vi "Realback2.vi"() -> ()   [LabVIEW 2013]
uses:
  <vilib>/Utility/file.llb/Write To Spreadsheet File (DBL).vi
  <vilib>/Utility/file.llb/Read From Spreadsheet File (DBL).vi
panel:
  out "Output array":dbl[][](array[numeric])=[[211.6, 0.38780028612303014], [211.60999999999999, 0.3845669527896967], [211.62, 0.3657997138769633], [211.63, 0.3474805436337587], [211.64, 0.32995436337624834], [211.65, 0.3122437768240314], [211.66, 0.2951436337625158], [211.67, 0.2787942775393399], [211.68, 0.2629261802575091], [211.69, 0.24712174535049974], [211.7, 0.23246380543633732], [211.71, 0.21756866952789733], [211.72, 0.2032354792560812], [211.73, 0.18945178826895767], [211.74, 0.17619527896995957], [211.75, 0.16343619456366493], [211.76, 0.1512828326180282], [211.77, 0.13936108726752736], [211.78, 0.12796037195994514], [211.79, 0.11670128755365022], [211.8, 0.10619170243204774], [211.81, 0.09626437768240538], [211.82, 0.08718154506437926], [211.82999999999998, 0.07816609442060239], [211.84, 0.06949399141631024], [211.85, 0.06115035765379196], [211.85999999999999, 0.05409570815450693], [211.87, 0.04653447782546495], [211.88, 0.040030901287553614], [211.89, 0.034256080114449174], [211.9, 0.028719027181688065], [211.91, 0.023262804005722462], [211.92, 0.019033476394849768], [211.93, 0.015508154506437763], [211.94, 0.011468955650929882], [211.95, 0.008281545064377656], [211.96, 0.005692417739628017], [211.97, 0.0037329041487839517], [211.98, 0.0022765379113018377], [211.99, 0.0005326180257510675], [212.0, 0.0005386266094420548], [212.01, 0.001001144492131604], [212.02, 0.0015979971387696558], [212.03, 0.0031499284692417515], [212.04, 0.004863090128755342], [212.05, 0.006630185979971357], [212.06, 0.009368669527896977], [212.07, 0.012598998569384807], [212.08, 0.016054649499284653], [212.09, 0.020632474964234614], [212.1, 0.0254995708154506], [212.11, 0.030854792560801106], [212.12, 0.037168669527896915], [212.13, 0.043395278969957006], [212.14000000000001, 0.050058226037196306], [212.15, 0.05790472103004361], [212.16, 0.06554334763948602], [212.17000000000002, 0.07354535050071673], [212.18, 0.08245851216023044], [212.19, 0.09229155937053117], [212.2, 0.10267010014306345], [212.21, 0.11381888412017369], [212.22, 0.12524005722460899], [212.23, 0.13723304721030297], [212.24, 0.14960200286123287], [212.25, 0.1625593705293301], [212.26, 0.17595951359084663], [212.27, 0.19006294706724108], [212.28, 0.2049556509299012], [212.29, 0.22014062947067292], [212.3, 0.23593648068669504], [212.31, 0.25293133047210187], [212.32, 0.27017496423461923], [212.33, 0.28806266094420385], [212.34, 0.30654978540772254], [212.35, 0.3253447782546466], [212.36, 0.34475236051501806], [212.37, 0.36438998569384445], [212.38, 0.3852260371959913], [212.39000000000001, 0.4064221745350483], [212.4, 0.42819256080114376]]
  in  "# of data rows":i32=91
  out "Voffset":dbl=6.2433 format="%_5g"
  out "Vtune":dbl=0.935 format="%_5g"
  out "Volts":dbl=3.245 format="%_4g"
  out "Temp C":dbl=24.12 format="%_4g"
  in  "# skip":i32
  in  "# of sweeps":i32=700
  out "Spectrum #":i32=699
  out "Chars":i32=494328
  out "Fcen":dbl=212.0 format="%#_13g"
  out "# Data points":i32=81
  in  "Offset V":dbl=0.032 format="%#_3g"
  out "NMR Graph + Fit":cluster{dbl, dbl}[](graph)=[{211.6, 0.38780028612303014}, {211.60999999999999, 0.3845669527896967}, {211.62, 0.3657997138769633}, {211.63, 0.3474805436337587}, {211.64, 0.32995436337624834}, {211.65, 0.3122437768240314}, {211.66, 0.2951436337625158}, {211.67, 0.2787942775393399}, {211.68, 0.2629261802575091}, {211.69, 0.24712174535049974}, {211.7, 0.23246380543633732}, {211.71, 0.21756866952789733}, {211.72, 0.2032354792560812}, {211.73, 0.18945178826895767}, {211.74, 0.17619527896995957}, {211.75, 0.16343619456366493}, {211.76, 0.1512828326180282}, {211.77, 0.13936108726752736}, {211.78, 0.12796037195994514}, {211.79, 0.11670128755365022}, {211.8, 0.10619170243204774}, {211.81, 0.09626437768240538}, {211.82, 0.08718154506437926}, {211.82999999999998, 0.07816609442060239}, {211.84, 0.06949399141631024}, {211.85, 0.06115035765379196}, {211.85999999999999, 0.05409570815450693}, {211.87, 0.04653447782546495}, {211.88, 0.040030901287553614}, {211.89, 0.034256080114449174}, {211.9, 0.028719027181688065}, {211.91, 0.023262804005722462}, {211.92, 0.019033476394849768}, {211.93, 0.015508154506437763}, {211.94, 0.011468955650929882}, {211.95, 0.008281545064377656}, {211.96, 0.005692417739628017}, {211.97, 0.0037329041487839517}, {211.98, 0.0022765379113018377}, {211.99, 0.0005326180257510675}, {212.0, 0.0005386266094420548}, {212.01, 0.001001144492131604}, {212.02, 0.0015979971387696558}, {212.03, 0.0031499284692417515}, {212.04, 0.004863090128755342}, {212.05, 0.006630185979971357}, {212.06, 0.009368669527896977}, {212.07, 0.012598998569384807}, {212.08, 0.016054649499284653}, {212.09, 0.020632474964234614}, {212.1, 0.0254995708154506}, {212.11, 0.030854792560801106}, {212.12, 0.037168669527896915}, {212.13, 0.043395278969957006}, {212.14000000000001, 0.050058226037196306}, {212.15, 0.05790472103004361}, {212.16, 0.06554334763948602}, {212.17000000000002, 0.07354535050071673}, {212.18, 0.08245851216023044}, {212.19, 0.09229155937053117}, {212.2, 0.10267010014306345}, {212.21, 0.11381888412017369}, {212.22, 0.12524005722460899}, {212.23, 0.13723304721030297}, {212.24, 0.14960200286123287}, {212.25, 0.1625593705293301}, {212.26, 0.17595951359084663}, {212.27, 0.19006294706724108}, {212.28, 0.2049556509299012}, {212.29, 0.22014062947067292}, {212.3, 0.23593648068669504}, {212.31, 0.25293133047210187}, {212.32, 0.27017496423461923}, {212.33, 0.28806266094420385}, {212.34, 0.30654978540772254}, {212.35, 0.3253447782546466}, {212.36, 0.34475236051501806}, {212.37, 0.36438998569384445}, {212.38, 0.3852260371959913}, {212.39000000000001, 0.4064221745350483}, {212.4, 0.42819256080114376}]
  out "File size (bytes)":i32=509277
  out "File name":string="C:\\Users\\plm\\Desktop\\rssmt\\NMR3521123599.xls"
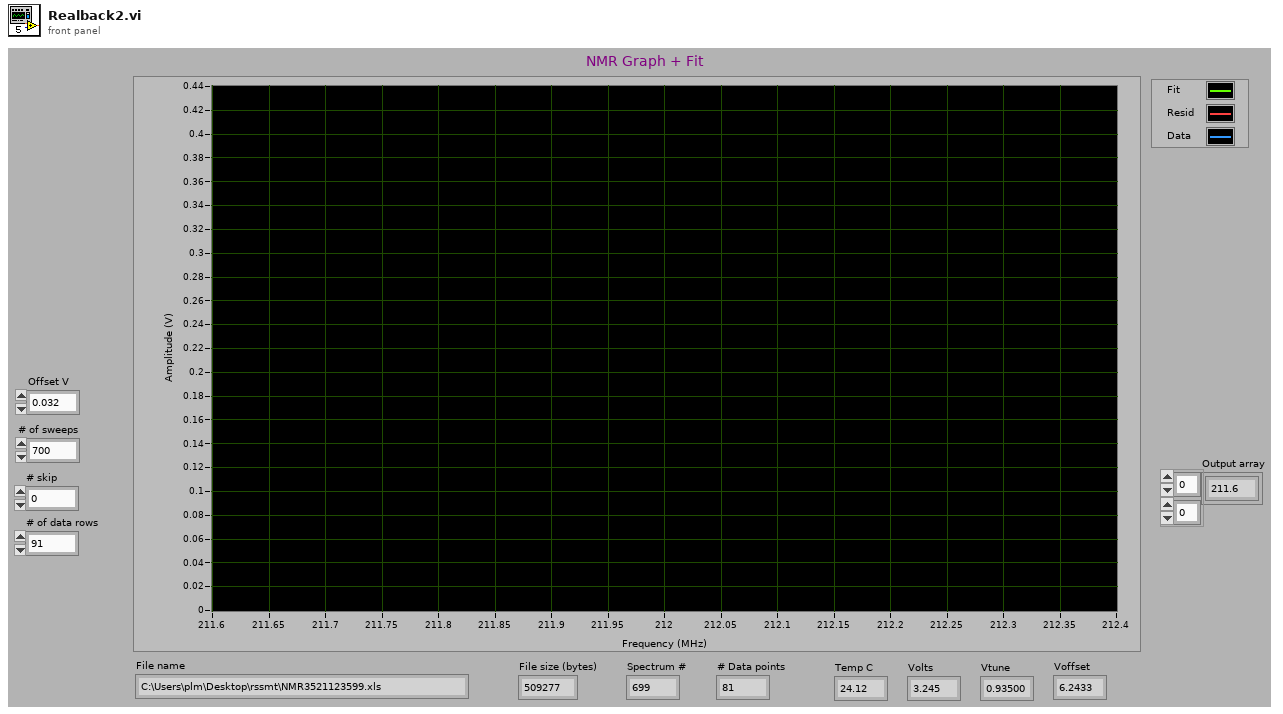
[diagram p1: front panel]
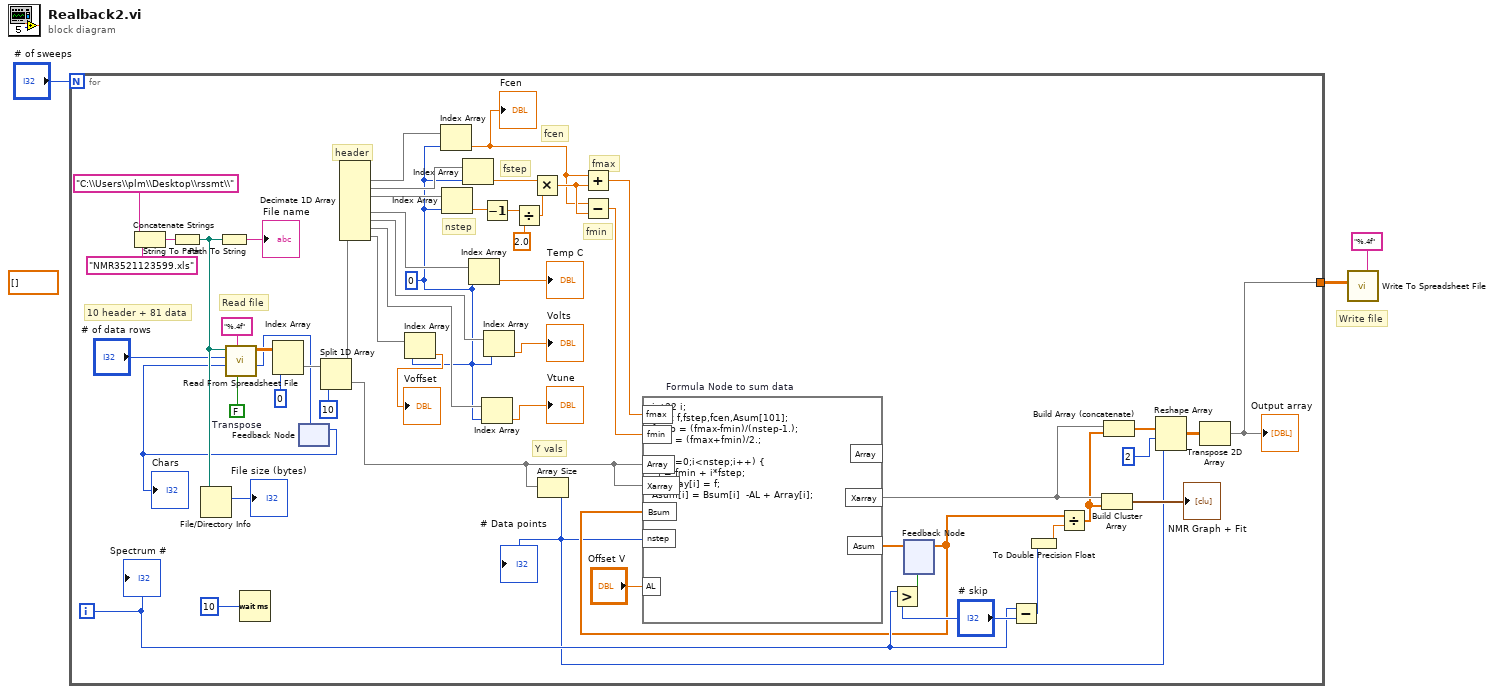
[diagram p0: block diagram]
diagram:
  (unwired) dbl[] []
  # "Write file"
  n1 = for {
    N: "# of sweeps" -> [_]
    tunnel: [w5] -> w1
    i -> [w26]
    w12 = 0
    w54 = FALSE  # Transpose
    # "10 header + 81 data"
    # "Read file"
    # "header"
    # "nstep"
    # "fstep"
    # "fcen"
    # "fmin"
    # "fmax"
    # "Y vals"
    n2 = Concatenate Strings "Concatenate Strings"("C:\\Users\\plm\\Desktop\\rssmt\\", "NMR3521123599.xls") -> (w57:string)
    n3 = String To Path(string=w57) -> (path=w53:path)
    n4 = File/Directory Info(path=w53) -> (size=→"File size (bytes)":i64)  [unwired: 1 in, 6 out]
    n5 = Path To String(path=w53) -> (string=→"File name":string)
    n6 = Wait (ms)(milliseconds to wait=10) -> ()  [unwired: 1 out]
    n7 = feedback #1() -> (w32:i32)  [unwired: 1 in]
    "Chars" <- w32
    n8 = call-poly <vilib>:"Read From Spreadsheet File.vi"("transpose (no:F)"=w54, "format (%.3f)"="%.4f", "start of read offset (chars.:0)"=w32, "number of rows (all:-1)"="# of data rows", "file path (dialog if empty)"=w53) -> ("mark after read (chars.)"=w33:i32, "all rows"=w48:dbl[][])  [unwired: 2 in, 3 out]
    n9 = Index Array "Index Array"(array=w48, index (col)=0) -> (element=w46:dbl[])  [unwired: 1 in]
    n10 = feedback-in #1(w33) -> ()
    n11 = Split 1D Array(array=w46, index=10) -> (first subarray=w49:dbl[], second subarray=w4:dbl[])
    n12 = Decimate 1D Array(w49) -> (w41:dbl[], w40:dbl[], w39:dbl[], w15:dbl[], w16:dbl[], w17:dbl[], w18:dbl[])  [unwired: 3 out]
    n13 = Index Array "Index Array"(array=w18, index=w12) -> (element=→"Voffset":dbl)
    n14 = Index Array "Index Array"(array=w41, index=w12) -> (element=w34:dbl)
    "Fcen" <- w34
    n15 = Index Array(array=w39, index=w12) -> (element=w37:dbl)
    n16 = Index Array(array=w40, index=w12) -> (element=w38:dbl)
    n17 = Index Array "Index Array"(array=w15, index=w12) -> (element=→"Temp C":dbl)
    n18 = Decrement(x=w37) -> (x-1=w45:dbl)
    n19 = Index Array "Index Array"(array=w17, index=w12) -> (element=→"Vtune":dbl)
    n20 = Index Array "Index Array"(array=w16, index=w12) -> (element=→"Volts":dbl)
    n21 = Divide(x=w45, y=2.0) -> (x/y=w43:dbl)
    n22 = Multiply(x=w38, y=w43) -> (x*y=w42:dbl)
    n23 = Array Size(array=w4) -> (size(s)=w7:i32)
    "# Data points" <- w7
    n24 = Add(x=w34, y=w42) -> (x+y=w23:dbl)
    n25 = Subtract(x=w34, y=w42) -> (x-y=w22:dbl)
    n26 = Greater?(x=w26, y="# skip") -> (0:w28:bool)
    n27 = feedback #2() -> (w13:dbl[])  [unwired: 1 in]
    n28 = formula code="int32 i;\nfloat f,fstep,fcen,Asum[101];\nfstep = (fmax-fmin)/(nstep-1.);\nfcen = (fmax+fmin)/2.;\n\nfor (i=0;i<nstep;i++) {\n  f = fmin + i*fstep;\n  Xarray[i] = f;\nAsum[i] = Bsum[i]  -AL + Array[i];\n}" "Formula Node to sum data"("nstep"=w7, "fmin"=w22, "fmax"=w23, "AL"="Offset V", "Array"=w4, "Xarray"=w4, "Bsum"=w13) -> ("Xarray"=w11:dbl[], "Asum"=w31:dbl[])  [unwired: 1 out]
    n29 = feedback-in #2(w31, w28) -> ()
    n30 = Subtract(x=w26, y="# skip") -> (x-y=w25:i32)
    n31 = To Double Precision Float(number=w25) -> (double precision float=w29:dbl)
    n32 = Divide(x=w13, y=w29) -> (x/y=w10:dbl[])
    n33 = Build Cluster Array ("Index & Bundle Cluster Array")(w11, w10) -> (→"NMR Graph + Fit":cluster{dbl, dbl}[])
    n34 = Build Array (concatenate)(w11, w10) -> (w9:dbl[])
    n35 = Reshape Array "Reshape Array"(w9, 2, w7) -> (w6:dbl[][])
    n36 = Transpose 2D Array(2D array=w6) -> (transposed array=w5:dbl[][])
    "Output array" <- w5
    "Spectrum #" <- w26
  }
  n37 = call-poly <vilib>:"Write To Spreadsheet File.vi"("format (%.3f)"="%.4f", "2D data"=w1) -> ()  [unwired: 6 in, 1 out]
